vi "UHR-Fleezers Control (host) - 11.9c.vi"() -> ()   [LabVIEW 2014] (continued)
            n1547 = call "IR AOM freq to word.vi"("Frequency In (MHz)"=w2214) -> ("Frequency Word Out (double)"=w2215:dbl)
            n1548 = To Quad Integer(1:w2215) -> (0:w2211:i64)
            n1549 = Add(x=w2210, y=w2211) -> (x+y=w2207:i64)
            n1550 = xnode "Read/Write Control"("FPGA VI Reference In"=w2209, "error in"=w2208, "FPGA TTrig Thresh"=w2207) -> ()  [unwired: 2 out]
          }
          frame #1 {
            "Threshold stored (nm)" <- w2219
          }
        }
      }
      event "FB Trig Integrate": Value Change {
        n1551 = event-data() -> ()  [unwired: 7 out]
        n1552 = local read "FB Trig Integrate"() -> (w2221:u32)
        n1553 = xnode "Read/Write Control"("FPGA VI Reference In"=w2223, "error in"=w2222, "FB Trig Integrate"=w2221) -> ("error out"=w2220:errorcluster)  [unwired: 1 out]
      }
      event "11": Value Change {
        n1554 = event-data() -> ()  [unwired: 7 out]
        n1555 = local read "11"() -> (w2224:bool)
        n1556 = case shown="True" w2224 {
          frame False {
          }
          frame True {
            n1557 = local read "Messages"() -> (w2226:string)
            n1558 = call "Update messages.vi"("Message to add"="You kicked it up to 11!", "Old message string"=w2226) -> ("New message string"=w2227:string)
            n1559 = call <vilib>:"Beep.vi"() -> ()  [unwired: 12 in]
            n1560 = local write "Messages"(w2227) -> ()
          }
        }
      }
      event "Trap Pos. FB ON": Value Change {
        n1561 = event-data() -> ()  [unwired: 7 out]
        n1562 = xnode "Read/Write Control"("FPGA VI Reference In"=w2230, "error in"=w2229, "Force feedback"="Trap Pos. FB ON") -> ()  [unwired: 2 out]
      }
      event "Remove Action Offset": Value Change {
        n1563 = event-data() -> ()  [unwired: 7 out]
        n1564 = local write "Remove Action Offset"(FALSE ("Remove Action Offset")) -> ()
        n1565 = local read "Trap Pos. FB Mult Factor"() -> (w2235:i64)
        n1566 = local read "Trap Pos FB Action"() -> (w2233:i64)
        n1567 = local read "Trap Pos. FB Offset Factor"() -> (w2231:i64)
        n1568 = Multiply(x=w2235, y=w2233) -> (x*y=w2234:i64)
        n1569 = Add(x=w2234, y=w2231) -> (x+y=w2232:i64)
        n1570 = local write "Trap Pos. FB Offset Factor"(w2232) -> ()
        n1571 = xnode "Read/Write Control"("FPGA VI Reference In"=w2238, "error in"=w2237, "Trap Pos. FB Offset Factor"=w2232) -> ()  [unwired: 2 out]
      }
      event "Remove Offset to factor": Value Change {
        n1572 = event-data() -> ()  [unwired: 7 out]
        n1573 = local write "Remove Offset to factor"(FALSE ("Remove Action Offset")) -> ()
        n1574 = local read "Trap Pos. FB Mult Factor"() -> (w2250:i64)
        n1575 = local read "Trap Pos FB Action"() -> (w2248:i64)
        n1576 = local read "Trap Pos. FB Offset Factor"() -> (w2247:i64)
        n1577 = Multiply(x=w2250, y=w2248) -> (x*y=w2249:i64)
        n1578 = local read "Trap Pos. FB Mult Factor"() -> (w2246:i64)
        n1579 = Add(x=w2249, y=w2247) -> (x+y=w2241:i64)
        n1580 = Multiply(x=32768, y="factor") -> (x*y=w2244:dbl)
        n1581 = Multiply(x=w2244, y=w2246) -> (x*y=w2245:dbl)
        n1582 = Subtract(x=w2241, y=w2245) -> (x-y=w2239:dbl)
        n1583 = To Quad Integer(1:w2239) -> (0:w2240:i64)
        n1584 = xnode "Read/Write Control"("FPGA VI Reference In"=w2253, "error in"=w2252, "Trap Pos. FB Offset Factor"=w2240) -> ()  [unwired: 2 out]
        n1585 = local write "Trap Pos. FB Offset Factor"(w2240) -> ()
      }
      event "Trap Pos. FB Range", "Trap Pos. FB Gains", "Trap Pos. FB Mult Factor", "Trap Pos. FB Offset Factor", "Trap Pos FB Negate Action", "Trap Pos FB Monitor\nT1 or T2", "Differential FB?", "Negate Diff?": Value Change {
        n1586 = event-data() -> ()  [unwired: 7 out]
        n1587 = local read "Negate Diff?"() -> (w2254:bool)
        n1588 = xnode "Read/Write Control"("FPGA VI Reference In"=w2264, "error in"=w2263, "Trap Pos. FB Range"="Trap Pos. FB Range", "Trap Pos. FB Gains"="Trap Pos. FB Gains", "Trap Pos. FB Mult Factor"="Trap Pos. FB Mult Factor", "Trap Pos. FB Offset Factor"="Trap Pos. FB Offset Factor", "Trap Pos FB Negate Action"="Trap Pos FB Negate Action", "Trap Pos FB Monitor T1 or T2"="Trap Pos FB Monitor\nT1 or T2", "AI1 X Scale"="Trap Pos. AI1 X Pre-scale", "Negate Diff?"=w2254, "Diff FB Measurement?"="Differential FB?") -> ()  [unwired: 2 out]
      }
      event "Trap Pos FB SP", "Trap Pos FB SP 2", "Use SP 2": Value Change {
        n1589 = event-data() -> ()  [unwired: 7 out]
        n1590 = Select(t="Trap Pos FB SP 2", s="Use SP 2", f="Trap Pos FB SP") -> (s? t:f=w2265:fxp<+/-,16,1>)
        n1591 = xnode "Read/Write Control"("FPGA VI Reference In"=w2270, "error in"=w2269, "Trap Pos. FB SP"=w2265) -> ()  [unwired: 2 out]
      }
      event "Offset SP2 from SP1": Value Change {
        n1592 = event-data() -> ()  [unwired: 7 out]
        n1593 = local read "Trap Pos FB SP"() -> (w2273:fxp<+/-,16,1>)
        n1594 = Add(x=w2273, y="SP2 Offset") -> (x+y=w2271:fxp<+/-,16,1>)
        n1595 = property on="Trap Pos FB SP 2" class="DigNum (strict)"("Val(Sgnl)"=w2271) -> ()  [unwired: 2 in, 2 out]
        n1596 = local write "Offset SP2 from SP1"(FALSE ("Offset SP2 from SP1")) -> ()
      }
      event "Set Reading to\nSetpoint": Value Change {
        # "This is the actual PID input signal"
        n1597 = event-data() -> ()  [unwired: 7 out]
        n1598 = local write "Set Reading to\nSetpoint"(FALSE ("Set SP to Reading")) -> ()
        n1599 = xnode "Read/Write Control"("FPGA VI Reference In"=w2279, "error in"=w2278) -> ("FPGA VI Reference Out"=w2277:T20, "error out"=w2276:errorcluster, "Trap Pos FB Int-Norm Signal"=w2275:fxp<+/-,16,1>)
        n1600 = local read "Differential FB?"() -> (w2280:bool)
        n1601 = case shown="False" w2280 {
          tunnel: [w2285 w2292] -> w2282
          tunnel: w2275 -> [w2283 w2292]
          frame False {
            n1602 = local read "Trap Pos FB Monitor\nT1 or T2"() -> (w2288:bool)
            n1603 = local read "Trap X AI1 (DMA)"() -> (w2291:T13)
            n1604 = Unbundle By Name(w2291) -> ("Set 1"=w2290:fxp<+/-,16,1>, "Set 2"=w2289:fxp<+/-,16,1>)
            n1605 = Select(t=w2290, s=w2288, f=w2289) -> (s? t:f=w2287:fxp<+/-,16,1>)
            n1606 = Not(x="Set SP Using...") -> (.not. x?=w2284:bool)
            n1607 = Select(t=w2283, s=w2284, f=w2287) -> (s? t:f=w2285:fxp<+/-,16,1>)
          }
          frame True {
          }
        }
        n1608 = xnode "Read/Write Control"("FPGA VI Reference In"=w2277, "error in"=w2276, "Trap Pos. FB SP"=w2282) -> ()  [unwired: 2 out]
        n1609 = local write "Trap Pos FB SP"(w2282) -> ()
      }
      event "Trap Pos. FB Out Scale 2^n": Value Change {
        n1610 = event-data() -> ()  [unwired: 7 out]
        n1611 = Scale By Power Of 2(n="Trap Pos. FB Out Scale 2^n", x=ext 1.0) -> (x*2^n=w2293:ext)
        n1612 = property on="Trap Pos. FB Mult Factor" class="DigNum (strict)"("Val(Sgnl)"=w2293) -> ()  [unwired: 2 in, 2 out]
      }
      event "Trap Pos FB Int Count": Value Change {
        n1613 = event-data() -> ()  [unwired: 7 out]
        n1614 = xnode "Read/Write Control"("FPGA VI Reference In"=w2298, "error in"=w2297, "Trap Pos FB Int Count"="Trap Pos FB Int Count") -> ()  [unwired: 2 out]
      }
      event "Trap pos": Value Change {
        n1615 = event-data() -> ()  [unwired: 7 out]
        n1616 = case shown="True" "Trap pos" {
          frame False {
            n1617 = property on="Trap Delta Graph" class="WFGraph (strict)"("Visible"=TRUE) -> ()  [unwired: 2 in, 2 out]
            n1618 = property on="Saved trap pos" class="WFGraph (strict)"("Visible"=FALSE) -> ()  [unwired: 2 in, 2 out]
          }
          frame True {
            n1619 = property on="Saved trap pos" class="WFGraph (strict)"("Visible"=TRUE) -> ()  [unwired: 2 in, 2 out]
            n1620 = property on="Trap Delta Graph" class="WFGraph (strict)"("Visible"=FALSE) -> ()  [unwired: 2 in, 2 out]
          }
        }
      }
      event "Save user params": Value Change {
        n1621 = event-data() -> ()  [unwired: 7 out]
        n1622 = local write "Save user params"(FALSE ("Save user\nparams")) -> ()
        n1623 = call "save control values.vi"("User"="User") -> ()  [unwired: 8 in, 1 out]
        n1624 = local read "Messages"() -> (w2310:string)
        n1625 = Concatenate Strings("User: ", "User", "\r", "Parameters saved.") -> (w2305:string)
        n1626 = call "Update messages.vi"("Message to add"=w2305, "Old message string"=w2310) -> ("New message string"=w2304:string)
        n1627 = local write "Messages"(w2304) -> ()
      }
      event "Load user params": Value Change {
        n1628 = event-data() -> ()  [unwired: 7 out]
        n1629 = local write "Load user params"(FALSE ("Read user\nparams")) -> ()
        n1630 = flat-sequence {
          tunnel: [w2342] -> w2330
          tunnel: [w2341] -> w2328
          tunnel: [w2340] -> w2326
          tunnel: [w2339] -> w2324
          tunnel: [w2338] -> w2322
          tunnel: [w2337] -> w2320
          tunnel: [w2336] -> w2318
          tunnel: [w2335] -> w2316
          tunnel: [w2334] -> w2314
          tunnel: [w2333] -> w2312
          tunnel: [w2352] -> w2331
          tunnel: w2330 -> [w2352]
          tunnel: [w2351] -> w2329
          tunnel: w2328 -> [w2351]
          tunnel: [w2350] -> w2327
          tunnel: w2326 -> [w2350]
          tunnel: [w2349] -> w2325
          tunnel: w2324 -> [w2349]
          tunnel: [w2348] -> w2323
          tunnel: w2322 -> [w2348]
          tunnel: [w2347] -> w2321
          tunnel: w2320 -> [w2347]
          tunnel: [w2346] -> w2319
          tunnel: w2318 -> [w2346]
          tunnel: [w2345] -> w2317
          tunnel: w2316 -> [w2345]
          tunnel: [w2344] -> w2315
          tunnel: w2314 -> [w2344]
          tunnel: [w2343] -> w2313
          tunnel: w2312 -> [w2343]
          tunnel: w2331 -> [w2369]
          tunnel: w2329 -> [w2368]
          tunnel: w2327 -> [w2367]
          tunnel: w2325 -> [w2366]
          tunnel: w2323 -> [w2365]
          tunnel: w2321 -> [w2364]
          tunnel: w2319 -> [w2363]
          tunnel: w2317 -> [w2362]
          tunnel: w2315 -> [w2361]
          tunnel: w2313 -> [w2360]
          frame #0 {
            # "Make exceptions.\nThese will not be\nloaded."
            n1631 = local read "Sample Channel\nFlow"() -> (w2337:bool)
            n1632 = local read "Green ON/Interlacing"() -> (w2338:bool)
            n1633 = local read "Trap 1 (ON/OFF)"() -> (w2342:bool)
            n1634 = local read "Trap 2 (ON/OFF)"() -> (w2341:bool)
            n1635 = local read "Trap Pos. FB ON"() -> (w2333:bool)
            n1636 = local read "Inject Pump 1"() -> (w2336:bool)
            n1637 = local read "Inject Pump 3"() -> (w2335:bool)
            n1638 = local read "Trap D (MHz)"() -> (w2334:dbl)
            n1639 = local read "Index"() -> (w2339:dbl)
            n1640 = local read "Fish"() -> (w2340:bool)
          }
          frame #1 {
            n1641 = local read "User"() -> (w2353:string)
            n1642 = call "retrieve control values.vi"("User"=w2353) -> ()  [unwired: 10 in, 1 out]
            n1643 = local read "Messages"() -> (w2359:string)
            n1644 = Concatenate Strings("User: ", w2353, "\r", "Parameters loaded.") -> (w2354:string)
            n1645 = call "Update messages.vi"("Message to add"=w2354, "Old message string"=w2359) -> ("New message string"=w2358:string)
            n1646 = local write "Messages"(w2358) -> ()
          }
          frame #2 {
            n1647 = local write "Sample Channel\nFlow"(w2364) -> ()
            n1648 = local write "Green ON/Interlacing"(w2365) -> ()
            n1649 = local write "Trap 1 (ON/OFF)"(w2369) -> ()
            n1650 = local write "Trap 2 (ON/OFF)"(w2368) -> ()
            n1651 = local write "Inject Pump 1"(w2363) -> ()
            n1652 = local write "Trap Pos. FB ON"(w2360) -> ()
            n1653 = local write "Inject Pump 3"(w2362) -> ()
            n1654 = local write "Trap D (MHz)"(w2361) -> ()
            n1655 = local write "Index"(w2366) -> ()
            n1656 = local write "Fish"(w2367) -> ()
          }
        }
      }
      event "Abort wiggle": Value Change {
        n1657 = event-data() -> ()  [unwired: 7 out]
        n1658 = flat-sequence {
          tunnel: w2373 -> [w2377]
          tunnel: w2372 -> [w2376]
          tunnel: [w2375] -> w2370
          tunnel: [w2379] -> w2371
          tunnel: w2370 -> [w2379]
          frame #0 {
            n1659 = xnode "Read/Write Control"("FPGA VI Reference In"=w2377, "error in"=w2376, "Abort wiggle 1"="Abort wiggle", "Abort wiggle 2"="Abort wiggle") -> ("error out"=w2375:errorcluster)  [unwired: 1 out]
          }
          frame #1 {
            n1660 = local write "Abort wiggle"(FALSE ("Abort wiggle")) -> ()
          }
        }
      }
    }
    "error out 2" <- w1158
    n1661 = node-c288() -> ()  [unwired: 2 out]
  }
  n1662 = node-c288() -> (w108:T22)  [unwired: 4 in]
  n1663 = local write "Target size"(cluster{"Width":dbl, "Height":dbl} {"Width"=40.0, "Height"=40.0} ("Target size")) -> ()
  n1664 = timed-loop "Run Scripts, including: stage motion" {
    tunnel: w113 -> [w2387]
    tunnel: w112 -> [w2388]
    tunnel: [w2388] -> w111
    tunnel: [w2387] -> w110
    timing: w108 -> [_]
    timing-out: [_] -> w107
    tunnel: w93 -> [w2386]
    tunnel: w94 -> [w2385]
    tunnel: w36 -> [w2382]
    tunnel: w35 -> [w2381]
    tunnel: w34 -> [w2383]
    tunnel: w33 -> [w2384]
    stop <- w2380 stop-if-true
    n1665 = node-c288() -> ()  [unwired: 1 in, 1 out]
    n1666 = event shown="[19] \"Take Detection Laser Image\": Value Change" {
      selector: _ -> [_ _ _ _ _ _ _ _ _ _ _ _ _ _ _ _ _ _ _ _ _]
      dyn-events: _ -> [_ _ _ _ _ _ _ _ _ _ _ _ _ _ _ _ _ _ _ _ _]
      timeout: _ -> [_ _ _ _ _ _ _ _ _ _ _ _ _ _ _ _ _ _ _ _ _]
      tunnel: ["Set Position" "Move to Position" _ _ "Read Harvard" _ _ _ _ _ _ _ "Got ADig bead" "Force FB Script" "Rupture Script" _ "Got DNA bead" "Take Stepping Data" _ "Take Detection Laser\nImage" _] -> _
      tunnel: [_ _ _ _ _ _ _ _ _ _ _ _ _ _ _ _ _ _ _ _ w3060] -> w2380
      tunnel: w2387 -> [w2406 w2414 w2427 w2457 _ w2505 w2545 w2628 w2659 w2793 w2819 w2854 _ w2871 _ _ _ _ _ _ _]
      tunnel: w2388 -> [w2407 w2415 w2428 w2458 _ w2506 w2546 w2629 w2660 w2794 w2820 w2855 _ w2872 _ _ _ _ _ _ _]
      tunnel: w2386 -> [_ _ _ _ w2490 _ _ _ _ _ _ _ _ _ _ _ _ _ _ _ _]
      tunnel: w2385 -> [_ _ _ _ w2489 _ _ _ _ _ _ _ _ _ _ _ _ _ _ _ _]
      tunnel: w2384 -> [_ _ _ _ _ _ _ _ _ _ _ _ _ _ _ _ _ _ _ _ _]
      tunnel: w2383 -> [_ _ _ _ _ _ _ _ _ _ _ _ _ _ _ _ _ _ _ _ _]
      tunnel: w2382 -> [_ _ _ _ _ _ _ _ _ _ _ _ _ _ _ _ _ _ _ _ _]
      tunnel: w2381 -> [_ _ _ _ _ _ _ _ _ _ _ _ _ _ _ _ _ _ _ _ _]
      event "Set Position", "Set Position 2", "Set Position 3", "Set Position 4", "Set Position 5", "Set Position 1": Value Change {
        n1667 = event-data() -> ()  [unwired: 1 in, 5 out]
        n1668 = Build Array("Set Position 1", "Set Position 2", "Set Position 3", "Set Position 4", "Set Position 5") -> (w2405:bool[])
        n1669 = Boolean Array To Number(Boolean array=w2405) -> (number=w2404:u32)
        n1670 = Logarithm Base 2(1:w2404) -> (0:w2396:dbl)
        n1671 = call "Read Stage Position.vi"("error in"=w2406, "VISA resource name in"=w2407) -> ("Current Position"=w2411:cluster{dbl, dbl, dbl}, "error out"=w2410:errorcluster)  [unwired: 2 out]
        n1672 = Decrement(x="Position") -> (x-1=w2394:dbl)
        n1673 = Greater Or Equal?(x=w2396, y=0.0) -> (x >= y?=w2397:bool)
        n1674 = Cluster To Array(cluster=w2411) -> (array=w2408:dbl[])
        n1675 = local write "Stage Control Serial Error"(w2410) -> ()
        n1676 = Select(t=w2396, s=w2397, f=w2394) -> (s? t:f=w2393:dbl)
        n1677 = Increment(x=w2393) -> (x+1=w2392:dbl)
        n1678 = Build Array (concatenate)(w2392, w2408) -> (w2391:dbl[])
        n1679 = Replace Array Subset(array="Saved Stage Positions", new element=w2391, index (row)=w2393) -> (w2409:dbl[][])  [unwired: 1 in]
        n1680 = local write "Saved Stage Positions"(w2409) -> ()
      }
      event "Move to Position": Value Change {
        n1681 = event-data() -> ()  [unwired: 1 in, 5 out]
        n1682 = flat-sequence {
          tunnel: w2415 -> [w2419]
          tunnel: w2414 -> [w2418]
          frame #0 {
            n1683 = local read "Saved Stage Positions"() -> (w2421:dbl[][])
            n1684 = local read "Position"() -> (w2420:dbl)
            n1685 = local write "Stage Moving"(TRUE ("Stage Moving")) -> ()
            n1686 = call "move to saved stage position.vi"("error in"=w2418, "Stage VISA resource name in"=w2419, "Position"=w2420, "Saved Stage Positions"=w2421) -> ("error out"=w2417:errorcluster)  [unwired: 1 out]
            n1687 = local write "Stage Control Serial Error"(w2417) -> ()
          }
          frame #1 {
            n1688 = call <vilib>:"Beep.vi"() -> ()  [unwired: 3 in, 9 out]
            n1689 = local write "Stage Moving"(FALSE ("Stage Moving")) -> ()
          }
        }
      }
      event "Move Cap. 1 (DNA Bottom)": Value Change {
        n1690 = event-data() -> ()  [unwired: 1 in, 5 out]
        n1691 = local write "Move Cap. 1 (DNA Bottom)"(FALSE ("Move Cap. 1 (DNA Right)")) -> ()
        n1692 = flat-sequence {
          tunnel: w2427 -> [w2430]
          tunnel: w2428 -> [w2431]
          tunnel: [w2431] -> w2425
          tunnel: [w2430] -> w2424
          tunnel: w2425 -> [w2433]
          tunnel: w2424 -> [w2432]
          frame #0 {
            n1693 = property on="Sample Channel\nFlow" class="Bool (strict)"("Val(Sgnl)"="Cap 1 Samp Flow ON") -> ()  [unwired: 2 in, 2 out]
          }
          frame #1 {
            n1694 = local read "Saved Stage Positions"() -> (w2443:dbl[][])
            n1695 = local write "Stage Moving"(TRUE ("Stage Moving")) -> ()
            n1696 = Array Subset(array=w2443, index (row)=0 ("index"), length (row)=1 ("length"), index (col)=1 ("index"), length (col)=3 ("length")) -> (w2440:dbl[][])
            n1697 = Reshape Array(w2440, 3 ("dimension size")) -> (w2438:dbl[])
            n1698 = Array To Cluster(array=w2438) -> (cluster=w2437:cluster{"[0]":dbl, "[1]":dbl, "[2]":dbl})
            n1699 = call "Set Stage Position.vi"("Position"=w2437, "error in"=w2432, "VISA resource name in"=w2433) -> ("error out"=w2436:errorcluster)  [unwired: 2 out]
            n1700 = local write "Stage Control Serial Error"(w2436) -> ()
          }
          frame #2 {
            n1701 = local write "Stage Moving"(FALSE ("Stage Moving")) -> ()
            n1702 = case shown="True" "Cap 1 Flow ON" {
              frame False {
              }
              frame True {
                n1703 = property on="Inject Pump 1" class="Bool (strict)"("Val(Sgnl)"=TRUE ("Value (Signaling)")) -> ()  [unwired: 2 in, 2 out]
              }
            }
            n1704 = call <vilib>:"Beep.vi"() -> ()  [unwired: 3 in, 9 out]
          }
          frame #3 {
            n1705 = property on="Sample Channel\nFlow" class="Bool (strict)"("Val(Sgnl)"=FALSE ("Value (Signaling)")) -> ()  [unwired: 2 in, 2 out]
            n1706 = local read "Cap. 2 BD T1?\n(ADig T1, DNA T2)"() -> (w2450:bool)
            n1707 = case shown="True" w2450 {
              tunnel: "Cap 1 T ON" -> [w2452 w2453]
              frame False {
                n1708 = property on="Trap 1 (ON/OFF)" class="Bool (strict)"("Val(Sgnl)"=w2452) -> ()  [unwired: 2 in, 2 out]
              }
              frame True {
                n1709 = property on="Trap 2 (ON/OFF)" class="Bool (strict)"("Val(Sgnl)"=w2453) -> ()  [unwired: 2 in, 2 out]
              }
            }
            n1710 = property on="Got DNA bead" class="Bool"("Key Focus"=TRUE) -> ()  [unwired: 2 in, 2 out]
          }
        }
      }
      event "Move Cap. 2 (ADig Top)": Value Change {
        n1711 = event-data() -> ()  [unwired: 1 in, 5 out]
        n1712 = local write "Move Cap. 2 (ADig Top)"(FALSE ("Move Cap. 2 (ADig Left)")) -> ()
        n1713 = flat-sequence {
          tunnel: w2457 -> [w2460]
          tunnel: w2458 -> [w2461]
          tunnel: [w2461] -> w2455
          tunnel: [w2460] -> w2454
          tunnel: w2455 -> [w2463]
          tunnel: w2454 -> [w2462]
          frame #0 {
            n1714 = property on="Sample Channel\nFlow" class="Bool (strict)"("Val(Sgnl)"="Cap 2 Samp Flow ON") -> ()  [unwired: 2 in, 2 out]
          }
          frame #1 {
            n1715 = local read "Saved Stage Positions"() -> (w2473:dbl[][])
            n1716 = local write "Stage Moving"(TRUE ("Stage Moving")) -> ()
            n1717 = Array Subset(array=w2473, index (row)=1 ("index"), length (row)=1 ("length"), index (col)=1 ("index"), length (col)=3 ("length")) -> (w2470:dbl[][])
            n1718 = disable-structure shown="Disabled" {
              frame Disabled {
                w2475 = FALSE ("Value (Signaling)")
                n1719 = property on="Trap 1 (ON/OFF)" class="Bool (strict)"("Val(Sgnl)"=w2475) -> ()  [unwired: 2 in, 2 out]
                n1720 = property on="Trap 1 (ON/OFF)" class="Bool (strict)"("Val(Sgnl)"=w2475) -> ()  [unwired: 2 in, 2 out]
              }
              frame Enabled {
              }
            }
            n1721 = Reshape Array(w2470, 3 ("dimension size")) -> (w2468:dbl[])
            n1722 = Array To Cluster(array=w2468) -> (cluster=w2467:cluster{"[0]":dbl, "[1]":dbl, "[2]":dbl})
            n1723 = call "Set Stage Position.vi"("Position"=w2467, "error in"=w2462, "VISA resource name in"=w2463) -> ("error out"=w2466:errorcluster)  [unwired: 2 out]
            n1724 = local write "Stage Control Serial Error"(w2466) -> ()
          }
          frame #2 {
            n1725 = local write "Stage Moving"(FALSE ("Stage Moving")) -> ()
            n1726 = call <vilib>:"Beep.vi"() -> ()  [unwired: 3 in, 9 out]
            n1727 = case shown="True" "Cap 2 Flow ON" {
              frame False {
              }
              frame True {
                n1728 = property on="Inject Pump 3" class="Bool (strict)"("Val(Sgnl)"=TRUE ("Value (Signaling)")) -> ()  [unwired: 2 in, 2 out]
              }
            }
          }
          frame #3 {
            n1729 = Wait (ms)(milliseconds to wait=u32 500) -> ()  [unwired: 1 out]
          }
          frame #4 {
            n1730 = local read "Cal @ (MHz)"() -> (w2481:dbl)
            n1731 = property on="Sample Channel\nFlow" class="Bool (strict)"("Val(Sgnl)"=FALSE ("Value (Signaling)")) -> ()  [unwired: 2 in, 2 out]
            n1732 = case shown="False" "Cap. 2 BD T1?\n(ADig T1, DNA T2)" {
              tunnel: "Cap 2 T ON" -> [w2486 w2487]
              frame False {
                n1733 = property on="Trap 2 (ON/OFF)" class="Bool (strict)"("Val(Sgnl)"=w2486) -> ()  [unwired: 2 in, 2 out]
              }
              frame True {
                n1734 = property on="Trap 1 (ON/OFF)" class="Bool (strict)"("Val(Sgnl)"=w2487) -> ()  [unwired: 2 in, 2 out]
              }
            }
            n1735 = property on="Got ADig bead" class="Bool"("Key Focus"=TRUE) -> ()  [unwired: 2 in, 2 out]
            n1736 = local write "Target"("Target\nON?") -> ()
            n1737 = property on="Trap D (MHz)" class="DigNum (strict)"("Val(Sgnl)"=w2481) -> ()  [unwired: 2 in, 2 out]
          }
        }
      }
      event "Read Harvard": Value Change {
        n1738 = event-data() -> ()  [unwired: 1 in, 5 out]
        n1739 = Concatenate Strings("write buffer", "\r") -> (w2492:string)
        n1740 = VISA Write(VISA resource name=w2490, write buffer=w2492, error in (no error)=w2489) -> (VISA resource name out=w2501:refnum<visa-resource-name>, error out=w2500:errorcluster)  [unwired: 1 out]
        n1741 = stacked-sequence {
          tunnel: [w2504] -> w2499
          tunnel: w2501 -> [w2504]
          tunnel: w2500 -> [w2503]
          tunnel: [w2503] -> w2494
          frame #0 {
            n1742 = Wait (ms)(milliseconds to wait=50) -> ()  [unwired: 1 out]
          }
        }
        n1743 = property class="Instr"(reference=w2499, error in=w2494) -> (reference out=w2498:refnum<visa-resource-name>, error out=w2496:errorcluster, "Serial Settings:Number of Bytes at Serial Port"=w2497:u32)
        "Serial Settings:Number of Bytes at Serial Port" <- w2497
        n1744 = VISA Read(VISA resource name=w2498, byte count=w2497, error in (no error)=w2496) -> (read buffer=w2495:string)  [unwired: 3 out]
        "read buffer" <- w2495
        n1745 = Fract/Exp String To Number(string=w2495) -> ()  [unwired: 5 out]
      }
      event "+z", "-z": Value Change {
        n1746 = event-data() -> ()  [unwired: 1 in, 5 out]
        n1747 = flat-sequence {
          tunnel: w2505 -> [w2527]
          tunnel: w2506 -> [w2507]
          frame #0 {
            n1748 = call "Read Stage Position.vi"("error in"=w2527, "VISA resource name in"=w2507) -> ("Current Position"=w2512:cluster{dbl, dbl, dbl}, "error out"=w2525:errorcluster, "VISA resource name out"=w2526:refnum<visa-resource-name>)  [unwired: 1 out]
            n1749 = local read "Saved Stage Positions"() -> (w2536:dbl[][])
            n1750 = Divide(x="z nudge increment (um)", y=1000.0) -> (x/y=w2524:dbl)
            n1751 = Boolean To (0,1)(Boolean="+z") -> (0, 1=w2516:i16)
            n1752 = Boolean To (0,1)(Boolean="-z") -> (0, 1=w2517:i16)
            n1753 = Array Subset(array=w2536, index (row)=1 ("index"), length (row)=1 ("length"), index (col)=1 ("index"), length (col)=3 ("length")) -> (w2533:dbl[][])
            n1754 = Multiply(x=w2516, y=w2524) -> (x*y=w2520:dbl)
            n1755 = Multiply(x=w2517, y=w2524) -> (x*y=w2518:dbl)
            n1756 = Unbundle(w2512) -> (w2510:dbl, w2509:dbl, w2513:dbl)
            n1757 = Negate(x=w2518) -> (-x=w2519:dbl)
            n1758 = Reshape Array(w2533, 3 ("dimension size")) -> (w2531:dbl[])
            n1759 = Add(x=w2520, y=w2519) -> (x+y=w2521:dbl)
            n1760 = Array To Cluster(array=w2531) -> ()  [unwired: 1 out]
            n1761 = Add(x=w2521, y=w2513) -> (x+y=w2511:dbl)
            n1762 = Bundle(cluster=w2512, w2510, w2509, w2511) -> (w2508:cluster{dbl, dbl, dbl})
            n1763 = call "Set Stage Position.vi"("Position"=w2508, "error in"=w2525, "VISA resource name in"=w2526) -> ("error out"=w2530:errorcluster)  [unwired: 2 out]
            n1764 = local write "Stage Moving"(TRUE ("Stage Moving")) -> ()
            n1765 = local write "Stage Control Serial Error"(w2530) -> ()
          }
          frame #1 {
            n1766 = local write "Stage Moving"(FALSE ("Stage Moving")) -> ()
            n1767 = call <vilib>:"Beep.vi"() -> ()  [unwired: 3 in, 9 out]
          }
        }
      }
      event "Cal/Data Acq. Spot": Value Change {
        n1768 = event-data() -> ()  [unwired: 1 in, 5 out]
        n1769 = flat-sequence {
          tunnel: w2545 -> [w2549]
          tunnel: w2546 -> [w2550]
          tunnel: [w2550] -> w2542
          tunnel: [w2549] -> w2541
          tunnel: w2542 -> [w2555]
          tunnel: w2541 -> [w2554]
          tunnel: ["Cal @ (MHz)"] -> w2539
          tunnel: [w2559] -> w2543
          tunnel: w2539 -> [w2559]
          tunnel: w2543 -> [w2570]
          tunnel: ["W/ Offset 1"] -> w2540
          tunnel: w2543 -> [w2591]
          tunnel: w2540 -> [w2589]
          frame #0 {
            n1770 = property on="Sample Channel\nFlow" class="Bool (strict)"("Val(Sgnl)"="Daq spot flow on") -> ()  [unwired: 2 in, 2 out]
            n1771 = Wait (ms)(milliseconds to wait=u32 250) -> ()  [unwired: 1 out]
          }
          frame #1 {
            n1772 = local read "Saved Stage Positions"() -> (w2552:dbl[][])
            n1773 = property on="Trap D (MHz)" class="DigNum (strict)"("Val(Sgnl)"="Cal @ (MHz)") -> ()  [unwired: 2 in, 2 out]
            n1774 = local write "Stage Moving"(TRUE ("Stage Moving")) -> ()
            n1775 = call "move to saved stage position.vi"("error in"=w2554, "Stage VISA resource name in"=w2555, "Position"="Cal Stage Position", "Saved Stage Positions"=w2552) -> ("error out"=w2553:errorcluster)  [unwired: 1 out]
            n1776 = local write "Stage Control Serial Error"(w2553) -> ()
          }
          frame #2 {
            n1777 = local write "Stage Moving"(FALSE ("Stage Moving")) -> ()
            n1778 = property on="Sample Channel\nFlow" class="Bool (strict)"("Val(Sgnl)"="Flow ON\nduring cal?") -> ()  [unwired: 2 in, 2 out]
            n1779 = call <vilib>:"Beep.vi"() -> ()  [unwired: 3 in, 9 out]
          }
          frame #3 {
            n1780 = local read "Wait Before Save (s)"() -> (w2562:u32)
            n1781 = Multiply(x=w2562, y=u32 1000 ("milliseconds to wait")) -> (x*y=w2563:u32)
            n1782 = Wait (ms)(milliseconds to wait=w2563) -> ()  [unwired: 1 out]
          }
          frame #4 {
            n1783 = property on="Save Calibration" class="Bool (strict)"("Val(Sgnl)"=TRUE ("Value (Signaling)")) -> ()  [unwired: 2 in, 2 out]
          }
          frame #5 {
            n1784 = Wait (ms)(milliseconds to wait=u32 2000) -> ()  [unwired: 1 out]
          }
          frame #6 {
            # "Check to see if \nsaving done"
            n1785 = while {
              stop <- w2566 stop-if-true
              n1786 = local read "Saving..."() -> (w2567:bool)
              n1787 = Wait (ms)(milliseconds to wait=u32 100) -> ()  [unwired: 1 out]
              n1788 = Not(x=w2567) -> (.not. x?=w2566:bool)
            }
          }
          frame #7 {
            n1789 = case shown="True" "W/ Offset 1" {
              tunnel: w2570 -> [_ w2571]
              frame False {
              }
              frame True {
                n1790 = stacked-sequence {
                  tunnel: w2571 -> [_ _ _ _ _ _ _ w2588]
                  frame #0 {
                    n1791 = property on="Trap D (MHz)" class="DigNum (strict)"("Val(Sgnl)"="Offset 1 Start (MHz)") -> ()  [unwired: 2 in, 2 out]
                    n1792 = Replace Array Subset(array=u32[] [0] ("Index Values"), new element="Offset 1 Set", index=0) -> (w2572:u32[])
                    n1793 = property on="Saved AOD Raster Scan Parameter Sets" class="Arr (strict)"("Index Values"=w2572) -> ()  [unwired: 2 in, 2 out]
                  }
                  frame #1 {
                    n1794 = Wait (ms)(milliseconds to wait=u32 200) -> ()  [unwired: 1 out]
                  }
                  frame #2 {
                    n1795 = property on="Load parameters" class="Bool (strict)"("Val(Sgnl)"=TRUE ("Value (Signaling)")) -> ()  [unwired: 2 in, 2 out]
                  }
                  frame #3 {
                    n1796 = Wait (ms)(milliseconds to wait=u32 200) -> ()  [unwired: 1 out]
                  }
                  frame #4 {
                    n1797 = property on="Trap Raster Scan" class="Bool (strict)"("Val(Sgnl)"=TRUE ("Value (Signaling)")) -> ()  [unwired: 2 in, 2 out]
                  }
                  frame #5 {
                    n1798 = Wait (ms)(milliseconds to wait=u32 2000) -> ()  [unwired: 1 out]
                  }
                  frame #6 {
                    n1799 = while {
                      stop <- w2585 stop-if-true
                      n1800 = local read "Raster Scanning..."() -> (w2587:bool)
                      n1801 = local read "Saving..."() -> (w2583:bool)
                      n1802 = Wait (ms)(milliseconds to wait=u32 100) -> ()  [unwired: 1 out]
                      n1803 = Not(x=w2583) -> (.not. x?=w2582:bool)
                      n1804 = Not(x=w2587) -> (.not. x?=w2584:bool)
                      n1805 = And(x=w2584, y=w2582) -> (x .and. y?=w2585:bool)
                    }
                  }
                  frame #7 {
                    n1806 = property on="Trap D (MHz)" class="DigNum (strict)"("Val(Sgnl)"=w2588) -> ()  [unwired: 2 in, 2 out]
                  }
                }
              }
            }
          }
          frame #8 {
            n1807 = local read "Save ave N"() -> (w2590:dbl)
            n1808 = case shown="False" "W/ Offset 2" {
              tunnel: w2591 -> [_ w2598]
              tunnel: w2590 -> [_ w2597]
              tunnel: w2589 -> [w2593 _]
              frame False {
                n1809 = case shown="False" w2593 {
                  frame False {
                    n1810 = Multiply(x="Cal read wait (s)", y=u32 1000 ("milliseconds to wait")) -> (x*y=w2595:u32)
                    n1811 = Wait (ms)(milliseconds to wait=w2595) -> ()  [unwired: 1 out]
                  }
                  frame True {
                  }
                }
              }
              frame True {
                n1812 = stacked-sequence {
                  tunnel: w2598 -> [_ _ _ _ _ _ _ _ _ w2619 _ _]
                  tunnel: w2597 -> [_ _ _ _ _ _ _ _ _ w2617 _ _]
                  frame #0 {
                    n1813 = property on="Save ave N" class="DigNum (strict)"("Val(Sgnl)"=1.0 ("Value (Signaling)")) -> ()  [unwired: 2 in, 2 out]
                  }
                  frame #1 {
                    n1814 = Wait (ms)(milliseconds to wait=u32 500) -> ()  [unwired: 1 out]
                  }
                  frame #2 {
                    n1815 = property on="Trap D (MHz)" class="DigNum (strict)"("Val(Sgnl)"="Offset 2 Start (MHz)") -> ()  [unwired: 2 in, 2 out]
                    n1816 = Replace Array Subset(array=u32[] [0] ("Index Values"), new element="Offset 2 Set", index=0) -> (w2603:u32[])
                    n1817 = property on="Saved AOD Raster Scan Parameter Sets" class="Arr (strict)"("Index Values"=w2603) -> ()  [unwired: 2 in, 2 out]
                  }
                  frame #3 {
                    n1818 = Wait (ms)(milliseconds to wait=u32 500) -> ()  [unwired: 1 out]
                  }
                  frame #4 {
                    n1819 = property on="Load parameters" class="Bool (strict)"("Val(Sgnl)"=TRUE ("Value (Signaling)")) -> ()  [unwired: 2 in, 2 out]
                  }
                  frame #5 {
                    n1820 = Wait (ms)(milliseconds to wait=u32 500) -> ()  [unwired: 1 out]
                  }
                  frame #6 {
                    n1821 = property on="Trap Raster Scan" class="Bool (strict)"("Val(Sgnl)"=TRUE ("Value (Signaling)")) -> ()  [unwired: 2 in, 2 out]
                  }
                  frame #7 {
                    n1822 = Wait (ms)(milliseconds to wait=u32 2000) -> ()  [unwired: 1 out]
                  }
                  frame #8 {
                    n1823 = while {
                      stop <- w2612 stop-if-true
                      n1824 = local read "Raster Scanning..."() -> (w2615:bool)
                      n1825 = local read "Saving..."() -> (w2613:bool)
                      n1826 = Wait (ms)(milliseconds to wait=u32 100) -> ()  [unwired: 1 out]
                      n1827 = Not(x=w2613) -> (.not. x?=w2611:bool)
                      n1828 = Not(x=w2615) -> (.not. x?=w2614:bool)
                      n1829 = And(x=w2614, y=w2611) -> (x .and. y?=w2612:bool)
                    }
                  }
                  frame #9 {
                    n1830 = property on="Trap D (MHz)" class="DigNum (strict)"("Val(Sgnl)"=w2619) -> ()  [unwired: 2 in, 2 out]
                    n1831 = property on="Saved AOD Raster Scan Parameter Sets" class="Arr (strict)"("Index Values"=u32[] [0]) -> ()  [unwired: 2 in, 2 out]
                    n1832 = property on="Save ave N" class="DigNum (strict)"("Val(Sgnl)"=w2617) -> ()  [unwired: 2 in, 2 out]
                  }
                  frame #10 {
                    n1833 = Wait (ms)(milliseconds to wait=u32 500) -> ()  [unwired: 1 out]
                  }
                  frame #11 {
                    n1834 = property on="Load parameters" class="Bool (strict)"("Val(Sgnl)"=TRUE ("Value (Signaling)")) -> ()  [unwired: 2 in, 2 out]
                  }
                }
              }
            }
          }
          frame #9 {
            n1835 = property on="Read Cal" class="Bool (strict)"("Val(Sgnl)"=TRUE ("Value (Signaling)")) -> ()  [unwired: 2 in, 2 out]
          }
          frame #10 {
            n1836 = Wait (ms)(milliseconds to wait=u32 1000) -> ()  [unwired: 1 out]
          }
          frame #11 {
            n1837 = property on="Fish" class="Bool (strict)"("Val(Sgnl)"=TRUE ("Value (Signaling)")) -> ()  [unwired: 2 in, 2 out]
          }
        }
        n1838 = local write "Cal/Data Acq. Spot"(FALSE ("Cal/Data Acq. Spot")) -> ()
      }
      event "Dump Beads": Value Change {
        n1839 = event-data() -> ()  [unwired: 1 in, 5 out]
        n1840 = flat-sequence {
          tunnel: ["Dump spot flow on?"] -> w2625
          tunnel: [w2637] -> w2626
          tunnel: w2625 -> [w2637]
          tunnel: w2629 -> [w2642]
          tunnel: w2628 -> [w2641]
          tunnel: [w2639] -> w2627
          tunnel: w2626 -> [w2639]
          tunnel: w2627 -> [w2653]
          frame #0 {
            w2630 = FALSE ("Value (Signaling)")
            n1841 = local read "Saving..."() -> (w2632:bool)
            n1842 = local write "Dump Beads"(FALSE ("Dump Beads")) -> ()
            n1843 = property on="Inject Pump 3" class="Bool (strict)"("Val(Sgnl)"=w2630) -> ()  [unwired: 2 in, 2 out]
            n1844 = property on="Inject Pump 1" class="Bool (strict)"("Val(Sgnl)"=w2630) -> ()  [unwired: 2 in, 2 out]
            n1845 = local write "Stop Saving"(w2632) -> ()
            n1846 = local write "Fish"(w2630) -> ()
          }
          frame #1 {
            w2633 = TRUE
            w2634 = FALSE ("Fl. Triggered...")
            n1847 = case shown="True" "Dump spot flow on?" {
              frame False {
              }
              frame True {
                n1848 = property on="Sample Channel\nFlow" class="Bool (strict)"("Val(Sgnl)"=TRUE ("Stage Moving")) -> ()  [unwired: 2 in, 2 out]
              }
            }
            n1849 = local write "Fl. Triggered..."(w2634) -> ()
            n1850 = local write "Tether"(w2634) -> ()
            n1851 = local write "Multiple tether"(w2634) -> ()
            n1852 = local write "Good tether"(w2634) -> ()
            n1853 = property on="Green ON/Interlacing" class="Bool (strict)"("Val(Sgnl)"=w2634) -> ()  [unwired: 2 in, 2 out]
            n1854 = property on="Trap Pos. FB ON" class="Bool (strict)"("Val(Sgnl)"=w2634) -> ()  [unwired: 2 in, 2 out]
            n1855 = property on="Trap Trig. Fl." class="Bool (strict)"("Val(Sgnl)"=w2634) -> ()  [unwired: 2 in, 2 out]
            n1856 = local write "Bad fit"(w2634) -> ()
            n1857 = local write "Hysteresis"(w2634) -> ()
            n1858 = property on="Fl. Triggered..." class="Bool (strict)"("Val(Sgnl)"=w2634) -> ()  [unwired: 2 in, 2 out]
            n1859 = local write "Restart DMA? (AOD)"(w2633) -> ()
            n1860 = local write "Save scans"(w2633) -> ()
            n1861 = property on="Dip for Protein" class="Bool (strict)"("Val(Sgnl)"=w2634) -> ()  [unwired: 2 in, 2 out]
            n1862 = property on="Pause dwell" class="Bool (strict)"("Val(Sgnl)"=w2634) -> ()  [unwired: 2 in, 2 out]
          }
          frame #2 {
            n1863 = property on="Trap Pos. FB Offset Factor" class="DigNum (strict)"("Val(Sgnl)"=i64 0 ("Value (Signaling)")) -> ()  [unwired: 2 in, 2 out]
          }
          frame #3 {
            n1864 = local read "Saved Stage Positions"() -> (w2643:dbl[][])
            n1865 = Array Subset(array=w2643, index (row)=3 ("index"), length (row)=1 ("length"), index (col)=1 ("index"), length (col)=3 ("length")) -> (w2648:dbl[][])
            n1866 = local write "Stage Moving"(TRUE ("Stage Moving")) -> ()
            n1867 = Reshape Array(w2648, 3 ("dimension size")) -> (w2646:dbl[])
            n1868 = Array To Cluster(array=w2646) -> (cluster=w2645:cluster{"[0]":dbl, "[1]":dbl, "[2]":dbl})
            n1869 = call "Set Stage Position.vi"("Position"=w2645, "error in"=w2641, "VISA resource name in"=w2642) -> ()  [unwired: 3 out]
          }
          frame #4 {
            w2654 = FALSE ("Value (Signaling)")
            n1870 = case shown="True" w2653 {
              frame False {
              }
              frame True {
                n1871 = property on="Sample Channel\nFlow" class="Bool (strict)"("Val(Sgnl)"=FALSE ("Stage Moving")) -> ()  [unwired: 2 in, 2 out]
              }
            }
            n1872 = property on="Trap 1 (ON/OFF)" class="Bool (strict)"("Val(Sgnl)"=w2654) -> ()  [unwired: 2 in, 2 out]
            n1873 = property on="Trap 2 (ON/OFF)" class="Bool (strict)"("Val(Sgnl)"=w2654) -> ()  [unwired: 2 in, 2 out]
            n1874 = call <vilib>:"Beep.vi"() -> ()  [unwired: 3 in, 9 out]
            n1875 = local write "Fish"(FALSE ("Fish for Tether")) -> ()
          }
          frame #5 {
            n1876 = property on="Move Cap. 2 (ADig Top)" class="Bool (strict)"("Val(Sgnl)"=TRUE ("Value (Signaling)")) -> ()  [unwired: 2 in, 2 out]
            n1877 = property on="Tab Control" class="TabCtl (strict)"("Val(Sgnl)"=T4."Status" ("Value (Signaling)")) -> ()  [unwired: 2 in, 2 out]
          }
        }
      }
      event "Dip for Protein": Value Change {
        n1878 = event-data() -> ()  [unwired: 1 in, 5 out]
        n1879 = case shown="True" "Dip for Protein" {
          tunnel: w2660 -> [_ w2662]
          tunnel: w2659 -> [_ w2661]
          frame False {
          }
          frame True {
            n1880 = while {
              tunnel: w2662 -> [w2673]
              tunnel: w2661 -> [w2672]
              i -> [w2668]
              stop <- w2663 stop-if-true
              n1881 = Increment(x=w2668) -> (x+1=→"Dip #":i32)
              n1882 = flat-sequence {
                tunnel: w2672 -> [w2684]
                tunnel: w2673 -> [w2685]
                tunnel: [w2685] -> w2677
                tunnel: [w2684] -> w2676
                tunnel: [w2678] -> w2664
                tunnel: [w2690] -> w2671
                tunnel: [w2691] -> w2670
                tunnel: w2677 -> [w2692]
                tunnel: w2676 -> [w2693]
                tunnel: [w2688] -> w2665
                tunnel: w2664 -> [w2688]
                tunnel: [w2701] -> w2675
                tunnel: w2671 -> [w2701]
                tunnel: [w2700] -> w2674
                tunnel: w2670 -> [w2700]
                tunnel: [w2697] -> w2669
                tunnel: [w2696] -> w2666
                tunnel: w2665 -> [w2696]
                tunnel: w2674 -> [w2721]
                tunnel: w2675 -> [w2722]
                tunnel: w2669 -> [w2723]
                tunnel: w2666 -> [w2720]
                tunnel: [w2782] -> w2663
                frame #0 {
                  n1883 = local read "Trap Pos. FB ON"() -> (w2678:bool)
                  n1884 = Compound Arithmetic op=AND("Flow ON\nduring dip?", "FB OFF when \nflow ON", w2678) -> (w2679:bool)
                  n1885 = case shown="True" "Move trap \nbefore dip move?" {
                    frame False {
                    }
                    frame True {
                      n1886 = property on="Trap D (MHz)" class="DigNum (strict)"("Val(Sgnl)"="Dipping D (MHz)") -> ()  [unwired: 2 in, 2 out]
                    }
                  }
                  n1887 = property on="Green ON/Interlacing" class="Bool (strict)"("Val(Sgnl)"="Green ON\nbefore dip?") -> ()  [unwired: 2 in, 2 out]
                  n1888 = property on="Sample Channel\nFlow" class="Bool (strict)"("Val(Sgnl)"="Flow ON\nduring dip?") -> ()  [unwired: 2 in, 2 out]
                  n1889 = case shown="True" w2679 {
                    frame False {
                    }
                    frame True {
                      n1890 = property on="Trap Pos. FB ON" class="Bool (strict)"("Val(Sgnl)"=FALSE ("Value (Signaling)")) -> ()  [unwired: 2 in, 2 out]
                    }
                  }
                }
                frame #1 {
                  n1891 = local read "Saved Stage Positions"() -> (w2695:dbl[][])
                  n1892 = local write "Cancel dwell"(FALSE ("Cancel dwell")) -> ()
                  n1893 = call "move to saved stage position.vi"("error in"=w2693, "Stage VISA resource name in"=w2692, "Position"="Dip Stage \nPosition", "Saved Stage Positions"=w2695) -> ("VISA resource name out"=w2690:refnum<visa-resource-name>, "error out"=w2691:errorcluster)
                }
                frame #2 {
                  n1894 = node-c288() -> (w2699:T22)  [unwired: 4 in]
                  n1895 = timed-loop {
                    timing: w2699 -> [_]
                    timing-out: [_] -> w2698
                    tunnel: [w2705] -> w2697
                    i -> [w2702]
                    stop <- w2706 stop-if-true
                    n1896 = node-c288() -> ()  [unwired: 1 in, 1 out]
                    n1897 = Greater Or Equal?(x=w2702, y="Dip Duration (s)") -> (x >= y?=w2714:bool)
                    n1898 = local read "Dip for Protein"() -> (w2707:bool)
                    n1899 = local read "Dump Beads"() -> (w2704:bool)
                    n1900 = local read "Cancel dwell"() -> (w2713:bool)
                    n1901 = local read "Pause dwell"() -> (w2710:bool)
                    n1902 = Not(x=w2707) -> (.not. x?=w2712:bool)
                    n1903 = Compound Arithmetic op=OR(w2713, w2714, w2712) -> (w2711:bool)
                    n1904 = Select(t=FALSE, s=w2710, f=w2711) -> (s? t:f=w2708:bool)
                    n1905 = Not(x=w2704) -> (.not. x?=w2703:bool)
                    n1906 = node-c288() -> ()  [unwired: 1 in, 1 out]
                    n1907 = And(x=w2707, y=w2703) -> (x .and. y?=w2705:bool)
                    n1908 = Or(x=w2708, y=w2704) -> (x .or. y?=w2706:bool)
                    "Dip Time (s)" <- w2702
                  }
                  n1909 = node-c288(w2698) -> ()  [unwired: 1 out]
                }
                frame #3 {
                  n1910 = case shown="True" w2723 {
                    tunnel: w2722 -> [_ w2728]
                    tunnel: w2721 -> [_ w2727]
                    tunnel: w2720 -> [_ w2724]
                    frame False {
                    }
                    frame True {
                      n1911 = flat-sequence {
                        tunnel: w2727 -> [w2732]
                        tunnel: w2728 -> [w2733]
                        tunnel: [w2733] -> w2726
                        tunnel: [w2732] -> w2725
                        tunnel: w2724 -> [w2729]
                        tunnel: w2726 -> [w2743]
                        tunnel: w2725 -> [w2742]
                        tunnel: w2724 -> [w2751]
                        frame #0 {
                          n1912 = local read "Sample Channel\nFlow"() -> (w2731:bool)
                          n1913 = case shown="True" w2731 {
                            tunnel: "Flow ON \nduring return\nfrom dip?" -> [w2734 w2737]
                            tunnel: w2729 -> [_ w2736]
                            frame False {
                              n1914 = case shown="True" w2734 {
                                frame False {
                                }
                                frame True {
                                n1915 = property on="Sample Channel\nFlow" class="Bool (strict)"("Val(Sgnl)"=TRUE ("Value (Signaling)")) -> ()  [unwired: 2 in, 2 out]
                                }
                              }
                            }
                            frame True {
                              n1916 = case shown="False" w2737 {
                                tunnel: w2736 -> [w2738 _]
                                frame False {
                                n1917 = property on="Trap Pos. FB ON" class="Bool (strict)"("Val(Sgnl)"=w2738) -> ()  [unwired: 2 in, 2 out]
                                n1918 = property on="Sample Channel\nFlow" class="Bool (strict)"("Val(Sgnl)"=FALSE ("Value (Signaling)")) -> ()  [unwired: 2 in, 2 out]
                                }
                                frame True {
                                }
                              }
                            }
                          }
                        }
                        frame #1 {
                          # "For turning on green laser before stage reaches lower spot"
                          n1919 = case shown="True" "Green ON\nafter start\nreturn?" {
                            frame False {
                            }
                            frame True {
                              n1920 = flat-sequence {
                                frame #0 {
                                n1921 = Multiply(x="Green delay after \nstart return (s)", y=1000.0) -> (x*y=w2748:dbl)
                                n1922 = Wait (ms)(milliseconds to wait=w2748) -> ()  [unwired: 1 out]
                                }
                                frame #1 {
                                n1923 = property on="Green ON/Interlacing" class="Bool (strict)"("Val(Sgnl)"=TRUE ("Value (Signaling)")) -> ()  [unwired: 2 in, 2 out]
                                }
                              }
                            }
                          }
                          n1924 = local read "Saved Stage Positions"() -> (w2746:dbl[][])
                          n1925 = local write "Cancel dwell"(FALSE ("Cancel dwell")) -> ()
                          n1926 = call "move to saved stage position.vi"("error in"=w2742, "Stage VISA resource name in"=w2743, "Position"="Return Stage \nPosition", "Saved Stage Positions"=w2746) -> ("error out"=w2744:errorcluster)  [unwired: 1 out]
                          n1927 = local write "Stage Control Serial Error"(w2744) -> ()
                        }
                        frame #2 {
                          n1928 = property on="Trap Pos. FB ON" class="Bool (strict)"("Val(Sgnl)"=w2751) -> ()  [unwired: 2 in, 2 out]
                          n1929 = case shown="True" "Green ON \nafter return?" {
                            frame False {
                            }
                            frame True {
                              n1930 = property on="Green ON/Interlacing" class="Bool (strict)"("Val(Sgnl)"=TRUE ("Value (Signaling)")) -> ()  [unwired: 2 in, 2 out]
                            }
                          }
                          n1931 = case shown="True" "Move trap after return?" {
                            frame False {
                            }
                            frame True {
                              n1932 = property on="Trap D (MHz)" class="DigNum (strict)"("Val(Sgnl)"="Dip Trap D 2 (MHz)") -> ()  [unwired: 2 in, 2 out]
                            }
                          }
                          n1933 = case shown="True" "Save data after return?" {
                            frame False {
                            }
                            frame True {
                              n1934 = property on="Start Saving" class="Bool (strict)"("Val(Sgnl)"=TRUE ("Value (Signaling)")) -> ()  [unwired: 2 in, 2 out]
                            }
                          }
                          n1935 = property on="Sample Channel\nFlow" class="Bool (strict)"("Val(Sgnl)"="Flow ON\nduring daq?") -> ()  [unwired: 2 in, 2 out]
                        }
                        frame #3 {
                          n1936 = node-c288() -> (w2760:T22)  [unwired: 4 in]
                          n1937 = timed-loop {
                            timing: w2760 -> [_]
                            timing-out: [_] -> w2759
                            i -> [w2761]
                            stop <- w2763 stop-if-true
                            n1938 = node-c288() -> ()  [unwired: 1 in, 1 out]
                            n1939 = local read "Dump Beads"() -> (w2762:bool)
                            n1940 = Greater Or Equal?(x=w2761, y="Dwell Duration (s)") -> (x >= y?=w2768:bool)
                            n1941 = local read "Dip for Protein"() -> (w2765:bool)
                            n1942 = Not(x=w2765) -> (.not. x?=w2764:bool)
                            n1943 = Compound Arithmetic op=OR(w2768, "Cancel dwell", w2764) -> (w2767:bool)
                            n1944 = node-c288() -> ()  [unwired: 1 in, 1 out]
                            n1945 = Select(t=FALSE, s="Pause dwell", f=w2767) -> (s? t:f=w2770:bool)
                            n1946 = Or(x=w2770, y=w2762) -> (x .or. y?=w2763:bool)
                            "Dwell Time (s)" <- w2761
                          }
                          n1947 = node-c288(w2759) -> ()  [unwired: 1 out]
                        }
                      }
                    }
                  }
                }
                frame #4 {
                  n1948 = local read "Dip for Protein"() -> (w2779:bool)
                  n1949 = local read "Tether"() -> (w2778:bool)
                  n1950 = local read "Dump Beads"() -> (w2780:bool)
                  n1951 = local write "Cancel dwell"(FALSE ("Cancel dwell")) -> ()
                  n1952 = Not(x=w2778) -> (.not. x?=w2777:bool)
                  n1953 = Not(x=w2779) -> (.not. x?=w2783:bool)
                  n1954 = Not(x="Cont. Repeat Dipping?") -> (.not. x?=w2785:bool)
                  n1955 = Compound Arithmetic op=OR(w2777, w2783, w2785, w2780) -> (w2782:bool)
                }
              }
            }
          }
        }
      }
      event "Profile": Value Change {
        n1956 = event-data() -> ()  [unwired: 1 in, 5 out]
        n1957 = flat-sequence {
          tunnel: w2794 -> [w2797]
          tunnel: w2793 -> [w2805]
          tunnel: [w2799] -> w2792
          tunnel: [w2798] -> w2791
          tunnel: [w2796] -> w2789
